vi "CPU Break Ref.vi"(8 "error in (no error)":errorcluster, 11 "Siemens Ctr":T1) -> (0 "error out":errorcluster, 3 "Siemens Ctr out":T1)   [LabVIEW 2014, in "Simatic S7.lvlib"]
uses:
  Simatic S7.lvlib
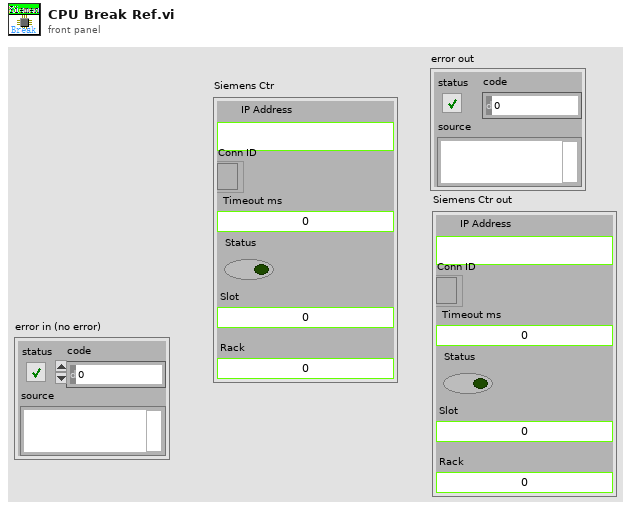
[diagram p1: front panel]
types:
  T1 = typedef "Simatic S7.lvlib/Siemens Ref.ctl" = cluster{"IP Address ":string, "Conn ID":refnum<k5>, "Timeout ms":i32, "Status":bool, "Slot":u16, "Rack":u16}
  T2 = typedef "Simatic S7.lvlib/Operation Siemens Ref.ctl" = enum16{"Init", "Add Ref", "Get Ref", "Set Error", "Close Close"}
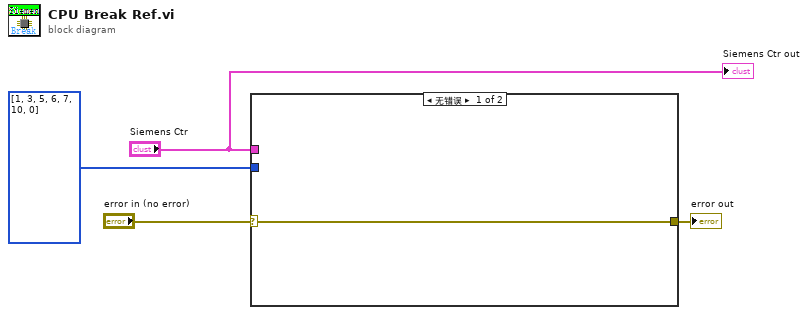
[diagram p0: block diagram]
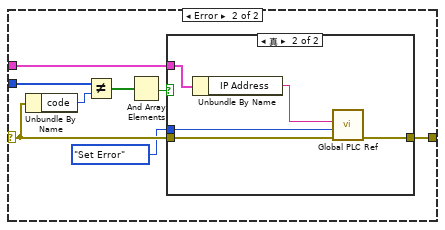
[diagram p2: hidden frame]
diagram:
  n1 = case shown="无错误" "error in (no error)" {
    selector: "error in (no error)" -> [w5 w10]
    tunnel: i32[] [1, 3, 5, 6, 7, 10, 0] ("[user-defined codes]") -> [_ w13]
    tunnel: "Siemens Ctr" -> [_ w7]
    tunnel: [w5 w6] -> w1
    frame No Error {
    }
    frame Error {
      n2 = Unbundle By Name(w10) -> ("code"=w12:i32)
      n3 = Not Equal?(x=w13, y=w12) -> (x != y?=w11:bool[])
      n4 = And Array Elements(Boolean array=w11) -> (logical AND=w9:bool)
      n5 = case shown="真" w9 {
        tunnel: w10 -> [w14 w19]
        tunnel: Operation_Siemens_Ref."Set Error" ("Operation Siemens Ref") -> [_ w18]
        tunnel: w7 -> [_ w17]
        tunnel: [w14 w15] -> w6
        frame False {
        }
        frame True {
          n6 = Unbundle By Name(w17) -> ("IP Address"=w16:string)
          n7 = call "Global PLC Ref.vi"("error in (no error)"=w19, "Operation Siemens Ref"=w18, "IP Address"=w16) -> ("error out"=w15:errorcluster)  [unwired: 4 in, 4 out]
        }
      }
    }
  }
  "error out" <- w1
  "Siemens Ctr out" <- "Siemens Ctr"
